vi "Publicador.vi"() -> ()   [LabVIEW 2018]
uses:
  RxTx/RxTx.lvclass
panel:
  in  "Publication":string
  in  "send":bool
  out "error out 2":errorcluster
  in  "Queue RX":refnum<class "RxTx.lvclass">
  in  "stop":bool
  # "PUB endpoint"
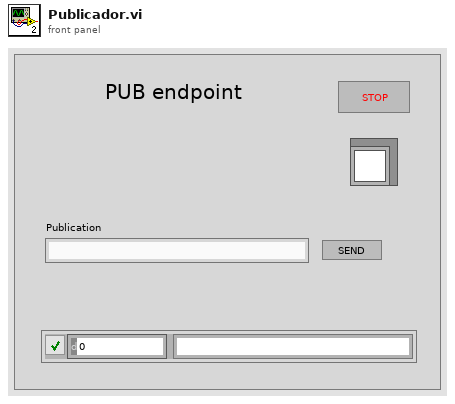
[diagram p1: front panel]
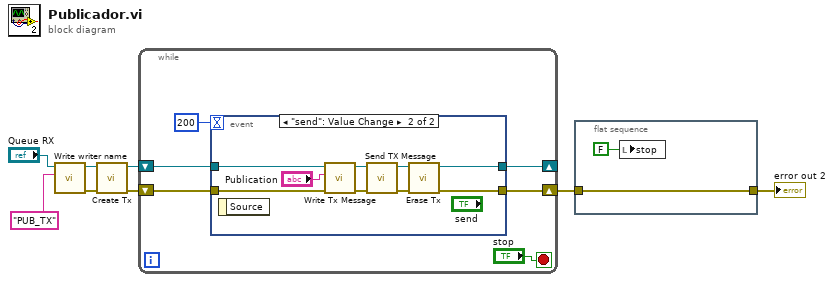
[diagram p0: block diagram]
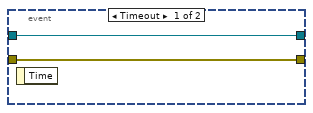
[diagram p2: hidden frame]
diagram:
  n1 = call-dynamic "Write writer name.vi"("Tx name"="PUB_TX", "RxTx in"="Queue RX") -> ("error out"=w5:errorcluster, "RxTx out"=w6:refnum<class "RxTx.lvclass">)  [unwired: 8 in]
  n2 = call "Create Tx.vi"("error in (no error)"=w5, "RxTx in"=w6) -> ("error out"=w4:errorcluster, "RxTx out"=w8:refnum<class "RxTx.lvclass">)  [unwired: 8 in]
  n3 = while {
    shift-right: [w11] -> _
    shift-left: w8 -> [w13]
    shift-right: [w10] -> w3
    shift-left: w4 -> [w12]
    stop <- "stop" stop-if-true
    n4 = event shown="[1] \"send\": Value Change" {
      selector: _ -> [_ _]
      dyn-events: _ -> [_ _]
      timeout: 200 -> [_ _]
      tunnel: [w16 w22] -> w11
      tunnel: [w15 w21] -> w10
      tunnel: w13 -> [w16 w18]
      tunnel: w12 -> [w15 w17]
      event Timeout {
        n5 = event-data() -> ()  [unwired: 1 in, 1 out]
      }
      event "send": Value Change {
        n6 = event-data() -> ()  [unwired: 1 in, 1 out]
        n7 = call "Write Tx Message.vi"("error in (no error)"=w17, "Tx Message"="Publication", "RxTx in"=w18) -> ("error out"=w19:errorcluster, "RxTx out"=w24:refnum<class "RxTx.lvclass">)  [unwired: 7 in]
        n8 = call "Send TX Message.vi"("error in (no error)"=w19, "RxTx in"=w24) -> ("error out"=w20:errorcluster, "RxTx out"=w23:refnum<class "RxTx.lvclass">)  [unwired: 8 in]
        n9 = call "Erase Tx.vi"("error in (no error)"=w20, "RxTx in"=w23) -> ("error out"=w21:errorcluster, "RxTx out"=w22:refnum<class "RxTx.lvclass">)  [unwired: 8 in]
      }
    }
  }
  n10 = flat-sequence {
    tunnel: w3 -> [w27]
    tunnel: [w27] -> w2
    frame #0 {
      n11 = local write "stop"(FALSE ("stop")) -> ()
    }
  }
  "error out 2" <- w2
